vi "Command (read) - AL.vi"(7 "timeout ms (100)":i32=100, 8 "error in (no error)":errorcluster, 10 "IP":string, 11 "connection ID in":refnum<k16>) -> (0 "error out":errorcluster, 2 "Alarm Code":string, 3 "connection ID out":refnum<k16>)   [LabVIEW 2016, in "SMD-7615.lvlib" / "eSCL.lvlib"]
doc: "AL - Alarm Code\nReads back an equivalent hexadecimal value of the Alarm Code’s 16-bit binary word."
uses:
  eSCL.lvlib
  String Command and Param.ctl
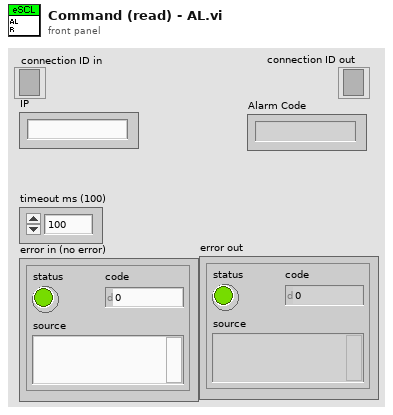
[diagram p1: front panel]
types:
  T1 = typedef "SMD-7615.lvlib/eSCL.lvlib/String Command and Param.ctl" = cluster{"Command":string, "String Parameler":string, "String Parameler Default":string}
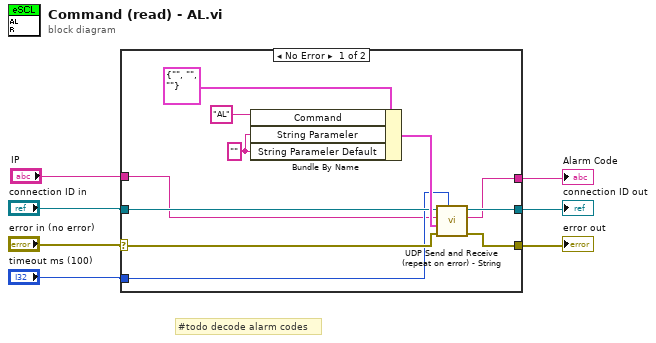
[diagram p0: block diagram]
diagram:
  # "#todo decode alarm codes"
  n1 = case shown="No Error" "error in (no error)" {
    selector: "error in (no error)" -> [w13 w19]
    tunnel: "connection ID in" -> [w11 w20]
    tunnel: [w16 w20] -> w2
    tunnel: [w14 w19] -> w3
    tunnel: "IP" -> [w9 _]
    tunnel: "timeout ms (100)" -> [w10 _]
    tunnel: [w15 _] -> w1
    frame No Error {
      w8 = "" ("String Parameler Default")
      n2 = Bundle By Name(cluster=T1 {"Command"="", "String Parameler"="", "String Parameler Default"=""} ("String Command & Param"), "Command"="AL", "String Parameler"=w8, "String Parameler Default"=w8) -> (w12:T1)
      n3 = call "UDP Send and Receive (repeat on error) - String.vi"("timeout ms (100)"=w10, "error in (no error)"=w13, "String Command & Param"=w12, "IP"=w9, "connection ID in"=w11) -> ("error out"=w14:errorcluster, "String Param out"=w15:string, "connection ID out"=w16:refnum<k16>)  [unwired: 4 in]
    }
    frame Error {
    }
  }
  "connection ID out" <- w2
  "error out" <- w3
  "Alarm Code" <- w1
